vi "Read HW Device Name.vi"(8 "error in (no error)":errorcluster, 11 "Analog in":refnum<class "Hardware.lvclass">) -> (0 "error out":errorcluster, 2 "Device Name":string, 3 "Analog out":refnum<class "Hardware.lvclass">)   [LabVIEW 2026, in "Hardware.lvlib" / "Hardware.lvclass"]
uses:
  Hardware.lvclass
  Hardware.lvclass/Hardware.ctl
  recovery/packages/oglib_file-4.0.1.22-8A89CE420A/File Group 0/user.lib/_OpenG.lib/file/file.llb/Strip Path Extension - String__ogtk.vi
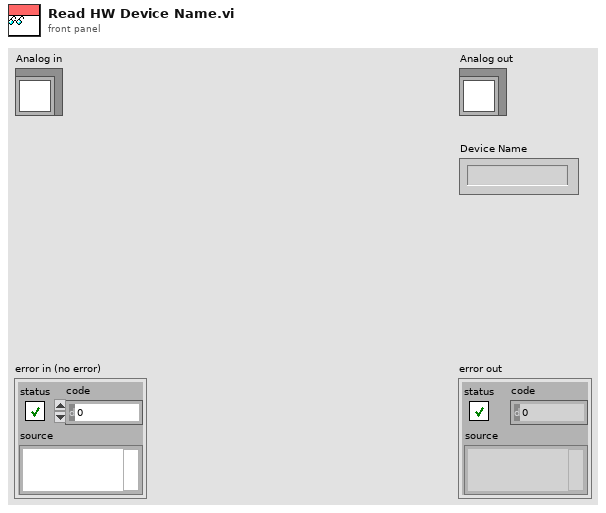
[diagram p1: front panel]
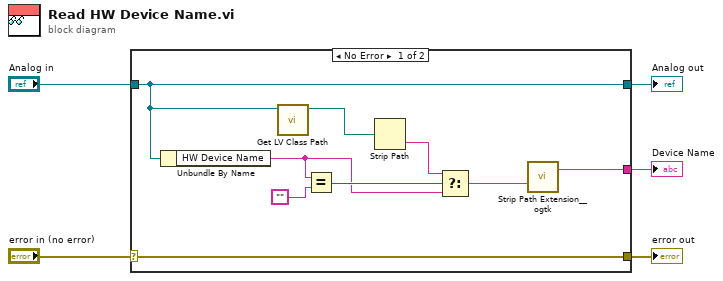
[diagram p0: block diagram]
diagram:
  n1 = case shown="No Error" "error in (no error)" {
    selector: "error in (no error)" -> [w14 w15]
    tunnel: [w14 w15] -> w4
    tunnel: [w8 w16] -> w2
    tunnel: "Analog in" -> [w8 w16]
    tunnel: [w6 _] -> w1
    frame No Error {
      n2 = Unbundle By Name(w8) -> ("HW Device Name"=w11:string)
      n3 = call <vilib>:"Get LV Class Path.vi"("object"=w8) -> ("class path"=w9:path)  [unwired: 9 in, 1 out]
      n4 = Equal?(x=w11, y="") -> (x = y?=w12:bool)
      n5 = Strip Path(path=w9) -> (name=w10:string)  [unwired: 1 out]
      n6 = Select(t=w10, s=w12, f=w11) -> (s? t:f=w7:string)
      n7 = call-poly "Strip Path Extension__ogtk.vi"("path"=w7) -> ("root"=w6:string)  [unwired: 1 out]
    }
    frame Error {
    }
  }
  "error out" <- w4
  "Analog out" <- w2
  "Device Name" <- w1
